vi "JFET_vs_GATE.vi"() -> ()   [LabVIEW 2018]
doc: "FET1 = I_DS vs V_GS\nMisura la caratteristica di un FET canale N\nfissando V sul DRAIN e variando V _GATE\nV_DRIAN puo' essere generata esternamente\nMisura la corrente utilizzando un OPAMP montato a transimpedenza sul SOURCE\nADL novembre 2019"
uses:
  <vilib>/DAQmx/write.llb/DAQmx Write (Analog DBL 1Chan 1Samp).vi
  <vilib>/DAQmx/create/channels.llb/DAQmx Create Channel (AO-Voltage-Basic).vi
  <vilib>/DAQmx/configure/timing.llb/DAQmx Timing (Sample Clock).vi
  <vilib>/DAQmx/miscellaneous.llb/DAQmx Fill In Error Info.vi
  <vilib>/Utility/file.llb/Write Delimited Spreadsheet (DBL).vi
panel:
  out "V_GATE":dbl=3.30078125 format="%_3g"
  in  "Fondo S. AI2":dbl(ring)=5.0 items=["10"=10.0, "5"=5.0, "0.5"=0.5, "0.05"=0.05]
  out "I_DS (mA)":dbl=46.1916015625 format="%_3f"
  in  "R_TRANSIMP (kOhm)":dbl=0.15 format="%_3g"
  in  "V_DRAIN":dbl=3.3 min=-10.0 max=10.0 step=0.025 format="%.3f"
  in  "Fondo S. AI1":dbl(ring)=10.0 items=["10"=10.0, "5"=5.0, "0.5"=0.5, "0.05"=0.05]
  in  "SALVA I DATI":bool=TRUE caption="ON\nOFF"
  out "V_DRAIN":dbl=3.3202880859375 format="%_3g"
  out "No Misura":i32=40
  in  "Fondo S. AI0":dbl(ring)=10.0 items=["10"=10.0, "5"=5.0, "0.5"=0.5, "0.05"=0.05]
  out "Corrente DRAIN-SOURCE in funzione della V_GS":cluster{dbl[], dbl[]}(graph)={[0.6005859375, 0.6689453125, 0.7373046875, 0.8056640625, 0.8789013671875, 0.947265625, 1.0156201171875, 1.083984375, 1.15234375, 1.220703125, 1.2939453125, 1.3623046875, 1.4306640625, 1.4990234375, 1.5673828125, 1.640625, 1.7089794921875, 1.77734375, 1.845703125, 1.9140576171875, 1.982421875, 2.0556640625, 2.1240234375, 2.1923828125, 2.2607421875, 2.3291015625, 2.40234375, 2.4706982421875, 2.5390625, 2.607421875, 2.67578125, 2.744140625, 2.8173876953125, 2.8857421875, 2.9541015625, 3.0224609375, 3.0908251953125, 3.1591796875, 3.232421875, 3.30078125], [-0.20615234375, -0.19925130208333333, -0.22102864583333337, -0.2377604166666667, -0.24801432291666667, -0.25559895833333335, -0.25872395833333334, -0.25888671875, -0.2591471354166667, -0.2592447916666667, -0.26002604166666665, -0.2601888020833334, -0.2601888020833334, -0.2602864583333333, -0.26005859375, -0.2582682291666667, -0.25374348958333337, -0.16917317708333335, -0.090234375, -0.03248697916666667, 0.0736328125, 0.158203125, 0.29300130208333336, 0.5859049479166667, 1.1076822916666667, 1.9851236979166669, 3.4820312500000004, 5.529947916666667, 8.339257812500001, 11.974967447916667, 17.2306640625, 22.196614583333336, 30.60947265625, 39.533365885416664, 48.62867838541667, 48.430338541666664, 47.899348958333334, 47.336979166666666, 46.7466796875, 46.1916015625]}
  out "V_OUT":dbl=-6.928740234375 format="%_3f"
  in  "# misure":i16=40
  in  "Vmax":dbl=3.3 max=100000.0
  in  "Vmin":dbl=0.6
  # "Valore consigliato  R_TRANSIMP = da 33 a 330 Ohm"
  # "1) Selezionare il valore minimo e massimo della tensione \napplicata al GATE  ed il n. di valori (equispaziati  tra gli estremi). \nSelezionare la tensione fissa applicata al DRAIN.\nSelezionare il valore della resistenza per TRANSIMPEDENZA."
  # "2) Collegamenti:\nAN.INPUT 0 (CB68) : CB22 e GATE\nAN.INPUT 1 (CB33) : Uscita OPAMP\nAN.INPUT 2 (CB65) : DRAIN\n    AL DRAIN VA COLLEGATO IL CB21 OPPURE IL     GENERATORE DI TENSIONE ESTERNO.  \nLa terra del circuito DEVE essere in comune alla terra della scheda (CB29)."
  # "3 ) Durante la misura gli indicatori mostrano i valori di I_DRAIN,   V_DRAIN , V_OUT ed il numero progressivo della misura.\nSul grafico viene mostrata la corrente che scorre da DRAIN a SOURCE  in funzione della tensione DRAIN-SOURCE."
  # "NO\nSI"
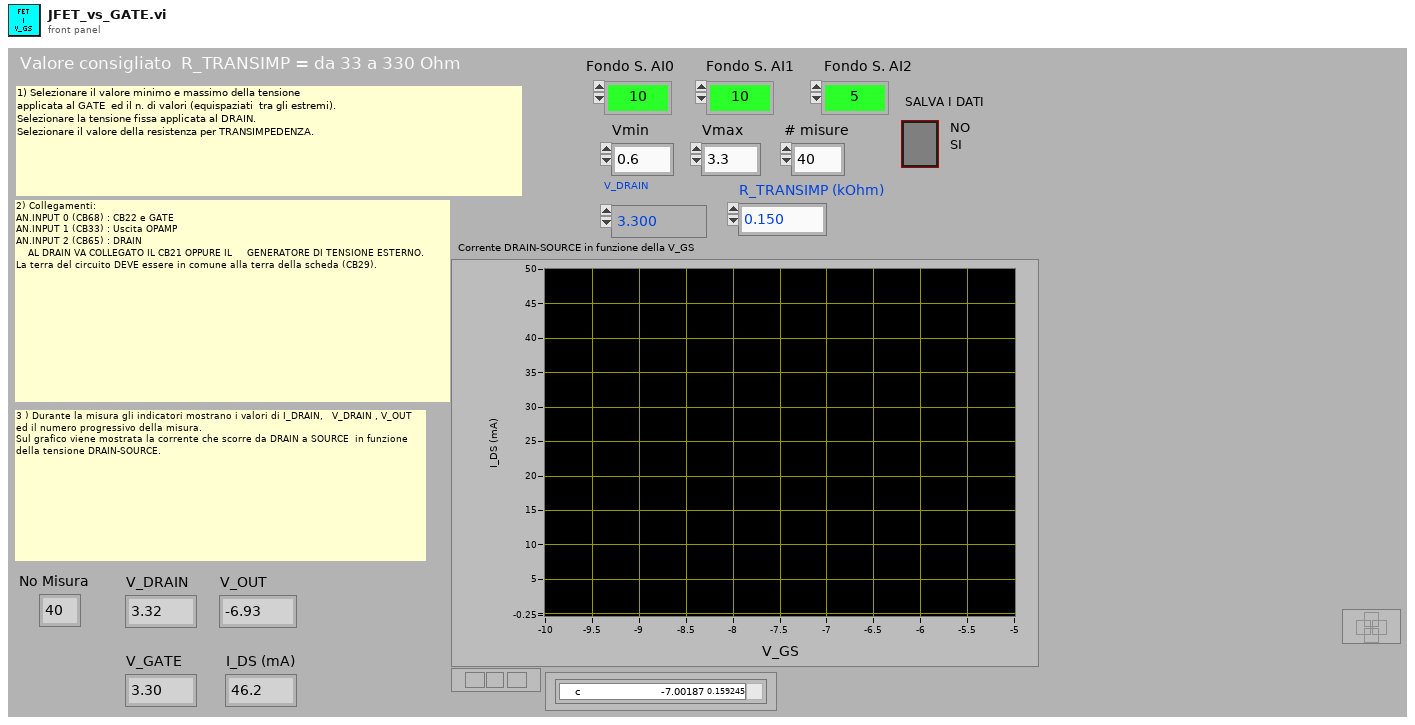
[diagram p1: front panel]
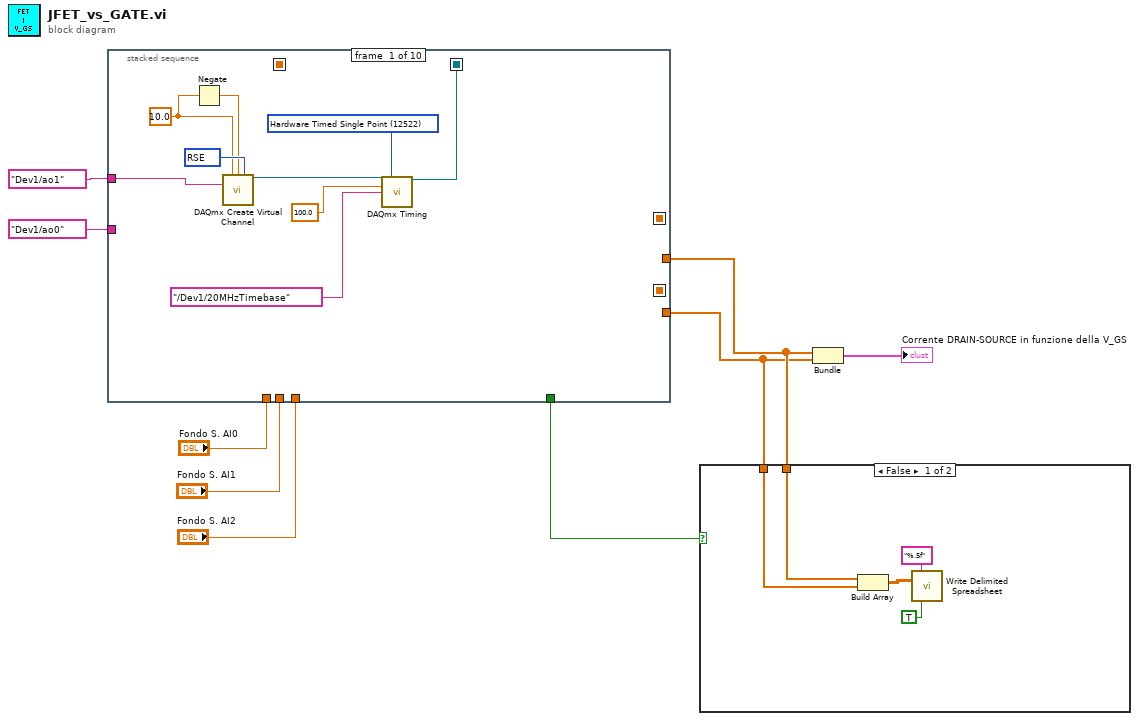
[diagram p0: block diagram]
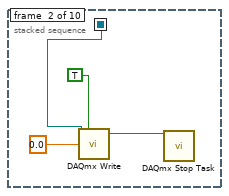
[diagram p3: hidden frame]
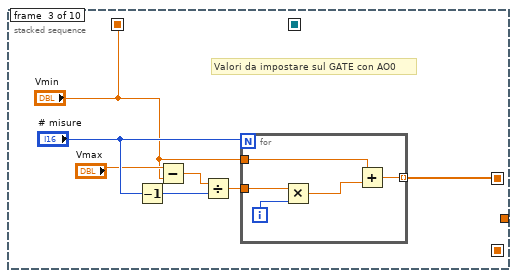
[diagram p4: hidden frame]
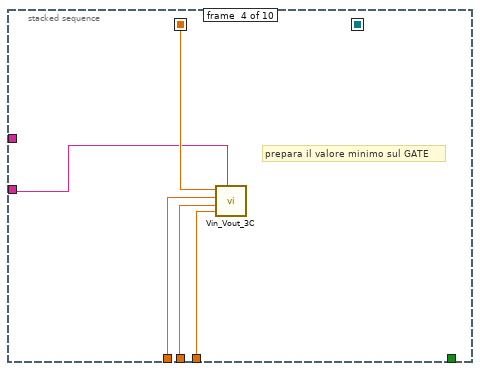
[diagram p5: hidden frame]
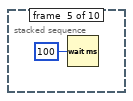
[diagram p6: hidden frame]
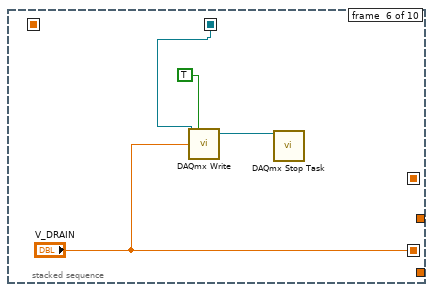
[diagram p7: hidden frame]
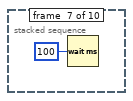
[diagram p8: hidden frame]
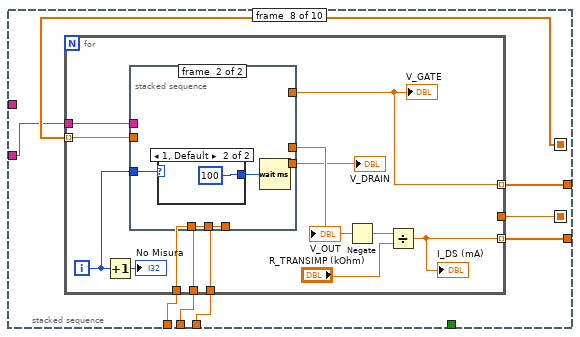
[diagram p9: hidden frame]
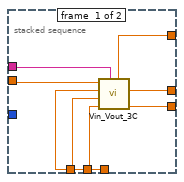
[diagram p10: hidden frame]
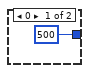
[diagram p11: hidden frame]
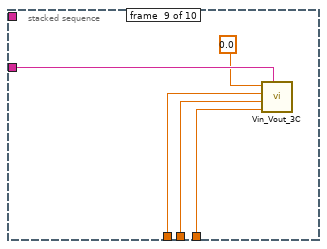
[diagram p12: hidden frame]
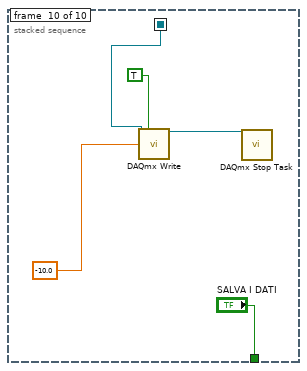
[diagram p13: hidden frame]
diagram:
  n1 = stacked-sequence {
    seq-local: [_ _ w26 _ _ _ _ _ _ _] -> [_ _ _ _ _ _ _ w52 _ _]
    seq-local: [w13 _ _ _ _ _ _ _ _ _] -> [_ w21 _ _ _ w43 _ _ _ w87]
    seq-local: [_ _ _ _ _ "V_DRAIN" _ _ _ _] -> [_ _ _ _ _ _ _ w47 _ _]
    seq-local: [_ _ "Vmin" _ _ _ _ _ _ _] -> [_ _ _ w37 _ _ _ _ _ _]
    tunnel: "Fondo S. AI1" -> [_ _ _ w38 _ _ _ w53 w82 _]
    tunnel: "Fondo S. AI0" -> [_ _ _ w39 _ _ _ w51 w83 _]
    tunnel: tag "Dev1/ao1" ("physical channels") -> [w12 _ _ _ _ _ _ _ _ _]
    tunnel: tag "Dev1/ao0" ("physical channels") -> [_ _ _ w35 _ _ _ w50 w81 _]
    tunnel: [_ _ _ _ _ _ _ w49 _ _] -> w3
    tunnel: [_ _ _ _ _ _ _ w48 _ _] -> w4
    tunnel: "Fondo S. AI2" -> [_ _ _ w36 _ _ _ w46 w79 _]
    tunnel: [_ _ _ _ _ _ _ _ _ "SALVA I DATI"] -> w1
    frame #0 {
      w17 = 12522 items=["Finite Samples"=10178, "Continuous Samples"=10123, "Hardware Timed Single Point"=12522] ("sample mode")
      w11 = 10.0 ("maximum value")
      w18 = 10083 items=["Default"=-1, "RSE"=10083, "Differential"=10106, "Pseudodifferential"=12529] ("output terminal configuration")
      n2 = Negate(x=w11) -> (-x=w10:dbl)
      n3 = call-poly <vilib>:"DAQmx Create Virtual Channel.vi"("maximum value"=w11, "minimum value"=w10, "output terminal configuration"=w18, "physical channels"=w12) -> ("task out"=w15:refnum<k21>)  [unwired: 5 in, 6 out]
      n4 = call-poly <vilib>:"DAQmx Timing.vi"("task/channels in"=w15, "sample mode"=w17, "rate"=100.0, "source"=tag "/Dev1/20MHzTimebase") -> ("task out"=w13:refnum<k21>)  [unwired: 3 in, 8 out]
    }
    frame #1 {
      n5 = call-poly <vilib>:"DAQmx Write.vi"("task/channels in"=w21, "auto start"=TRUE, "data"=0.0) -> ("task out"=w20:refnum<k21>)  [unwired: 1 in, 11 out]
      n6 = call <vilib>:"DAQmx Stop Task.vi"("task/channels in"=w20) -> ()  [unwired: 1 in, 14 out]
    }
    frame #2 {
      # "Valori da impostare sul GATE con AO0"
      n7 = Decrement(x="# misure") -> (x-1=w28:i16)
      n8 = Subtract(x="Vmax", y="Vmin") -> (x-y=w29:dbl)
      n9 = Divide(x=w29, y=w28) -> (x/y=w27:dbl)
      n10 = for {
        N: "# misure" -> [_]
        tunnel: "Vmin" -> [w34]
        tunnel: [w33] -> w26 mode=indexing
        tunnel: w27 -> [w32]
        i -> [w31]
        n11 = Multiply(x=w32, y=w31) -> (x*y=w30:dbl)
        n12 = Add(x=w34, y=w30) -> (x+y=w33:dbl)
      }
    }
    frame #3 {
      # "prepara il valore minimo sul GATE"
      n13 = call "Vin_Vout_3C.vi"("Canale uscita"=w35, "Fondo Scala AI2 (65)"=w36, "Fondo Scala AI1 (33)"=w38, "Fondo Scala AI0 (68)"=w39, "V in volt"=w37) -> ()  [unwired: 6 out]
    }
    frame #4 {
      n14 = Wait (ms)(milliseconds to wait=u32 100) -> ()  [unwired: 1 out]
    }
    frame #5 {
      n15 = call-poly <vilib>:"DAQmx Write.vi"("task/channels in"=w43, "auto start"=TRUE, "data"="V_DRAIN") -> ("task out"=w42:refnum<k21>)  [unwired: 1 in, 11 out]
      n16 = call <vilib>:"DAQmx Stop Task.vi"("task/channels in"=w42) -> ()  [unwired: 1 in, 14 out]
    }
    frame #6 {
      n17 = Wait (ms)(milliseconds to wait=u32 100) -> ()  [unwired: 1 out]
    }
    frame #7 {
      n18 = for {
        tunnel: w52 -> [w60] mode=indexing
        tunnel: w53 -> [w66]
        tunnel: w51 -> [w64]
        tunnel: w50 -> [w62]
        tunnel: [w59] -> w49 mode=indexing
        tunnel: [w54] -> w48 mode=indexing
        tunnel: w47 -> [_]
        tunnel: w46 -> [w58]
        i -> [w63]
        n19 = Increment(x=w63) -> (x+1=→"No Misura":i32)
        n20 = stacked-sequence {
          tunnel: w60 -> [w73 _]
          tunnel: w66 -> [w71 _]
          tunnel: w64 -> [w72 _]
          tunnel: w63 -> [_ w75]
          tunnel: w62 -> [w74 _]
          tunnel: w58 -> [w70 _]
          tunnel: [w69 _] -> w54
          tunnel: [w68 _] -> w57
          tunnel: [w67 _] -> w55
          frame #0 {
            n21 = call "Vin_Vout_3C.vi"("Canale uscita"=w74, "Fondo Scala AI2 (65)"=w70, "Fondo Scala AI1 (33)"=w71, "Fondo Scala AI0 (68)"=w72, "V in volt"=w73) -> ("V2 medio"=w67:dbl, "V1 medio"=w68:dbl, "V0 medio"=w69:dbl)  [unwired: 3 out]
          }
          frame #1 {
            n22 = case shown="1, Default" w75 {
              tunnel: [500 u32 100 ("milliseconds to wait")] -> w76
              frame 0 {
              }
              frame 1, Default {
              }
            }
            n23 = Wait (ms)(milliseconds to wait=w76) -> ()  [unwired: 1 out]
          }
        }
        "V_OUT" <- w57
        "V_DRAIN" <- w55
        "V_GATE" <- w54
        n24 = Negate(x=w57) -> (-x=w56:dbl)
        n25 = Divide(x=w56, y="R_TRANSIMP (kOhm)") -> (x/y=w59:dbl)
        "I_DS (mA)" <- w59
      }
    }
    frame #8 {
      n26 = call "Vin_Vout_3C.vi"("Canale uscita"=w81, "Fondo Scala AI2 (65)"=w79, "Fondo Scala AI1 (33)"=w82, "Fondo Scala AI0 (68)"=w83, "V in volt"=0.0) -> ()  [unwired: 6 out]
    }
    frame #9 {
      n27 = call-poly <vilib>:"DAQmx Write.vi"("task/channels in"=w87, "auto start"=TRUE, "data"=-10.0) -> ("task out"=w85:refnum<k21>)  [unwired: 1 in, 11 out]
      n28 = call <vilib>:"DAQmx Stop Task.vi"("task/channels in"=w85) -> ()  [unwired: 1 in, 14 out]
    }
  }
  n29 = case shown="False" w1 {
    tunnel: w4 -> [w93 _]
    tunnel: w3 -> [w92 _]
    frame False {
      n30 = Build Array(w93, w92) -> (w89:dbl[][])
      n31 = call-poly <vilib>:"Write Delimited Spreadsheet.vi"("format (%.3f)"="%.5f", "2D data"=w89, "transpose? (no:F)"=TRUE) -> ()  [unwired: 11 in, 2 out]
    }
    frame True {
    }
  }
  n32 = Bundle(w4, w3) -> (→"Corrente DRAIN-SOURCE in funzione della V_GS":cluster{dbl[], dbl[]})  [unwired: 1 out]
